vi "CreatSendArray.vi"(0 "AngleSample":dbl[](array[numeric]), 4 "AxisForces":dbl[](array[numeric]), 6 "AccumulateSample":dbl[](array[numeric]), 7 "数组":dbl[](array[numeric]), 8 "DisplacementSample":dbl[](array[numeric]), 9 "ControlOutput":dbl[](array[numeric]), 10 "TorqueSampledata":dbl[](array[numeric]), 11 "Command":dbl[](array[numeric])) -> (3 "SendArray":dbl[](array[numeric]))   [LabVIEW 2014]
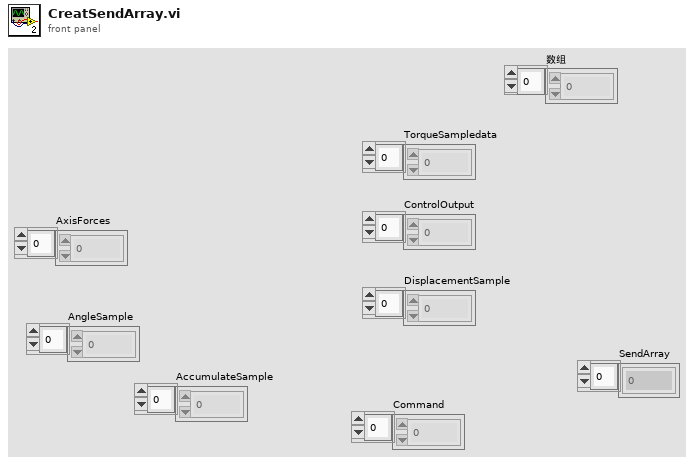
[diagram p1: front panel]
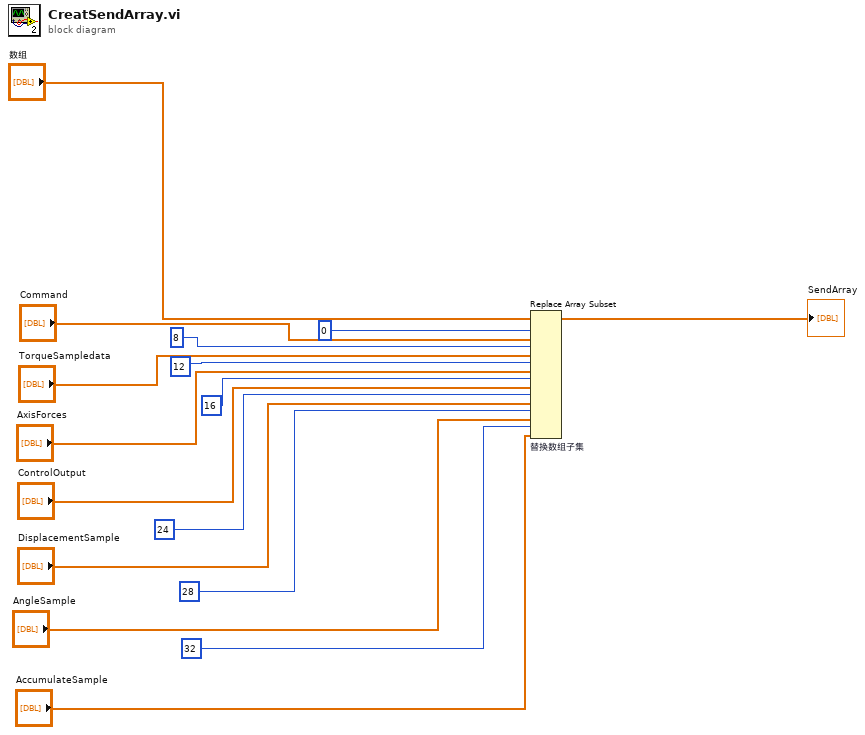
[diagram p0: block diagram]
diagram:
  n1 = Replace Array Subset "替换数组子集"(array="数组", new element #1="Command", index #1=0 ("index"), new element #2="TorqueSampledata", index #2=8 ("index"), new element #3="AxisForces", index #3=12 ("index"), new element #4="ControlOutput", index #4=16 ("index"), new element #5="DisplacementSample", index #5=24 ("index"), new element #6="AngleSample", index #6=28 ("index"), new element #7="AccumulateSample", index #7=32 ("index")) -> (→"SendArray":dbl[])
